vi "Main.vi"(10 "JQMHStartup":refnum<class "ModuleStartup.lvclass">, 11 "SingleLoopTemplate in":refnum<class "Metronome.lvclass">) -> ()   [LabVIEW 2024, in "Metronome.lvclass"]
uses:
  Metronome.lvclass
  C:/Git/JA/JQMH/RQMHCore/ModuleCore/Module.lvclass
  RQMHCore/Startup/ModuleStartup.lvclass
  RQMHCore/ModuleCore/Module.lvclass/Module.ctl
  RQMHCore/ActionStack/Stack/Stack.lvclass/Stack.ctl
  RQMHCore/ActionStack/Stack/Stack.lvclass
  Metronome.lvclass/Metronome.ctl
  C:/Git/JA/JQMH/ModuleTemplates/Metronome/Metronome.lvclass
  RQMHCore/ModuleCore/Module.lvclass
  RQMHCore/ModuleCore/Reply.ctl
  <vilib>/Utility/miscctls.llb/LVPointTypeDef.ctl
  RQMHCore/ModuleCore/InitialiseReplyArgs.ctl
  RQMHCore/ActionStack/Stack/StackFromSingleWithPayload.vi
  RQMHCore/ActionStack/Stack/InitFromString.vi
  RQMHCore/ActionStack/Stack/AppendStacks.vi
  Do Something Args.ctl
panel:
  out "period (ms)":u32
  out "error out":errorcluster
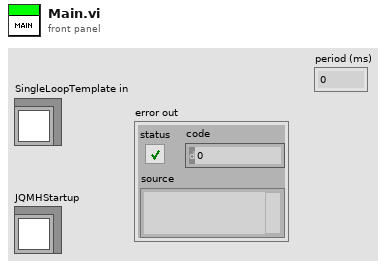
[diagram p1: front panel]
types:
  T1 = typedef "Metronome.lvclass/Request Events--cluster.ctl" = cluster{"Do Something":refnum<user-event>}
  T2 = cluster{"StandardRequests":refnum<event-registration>, "Event Registration Refnum":refnum<event-registration>}
  T3 = cluster{"Module":refnum<class "Metronome.lvclass">, "Args":string}
  T4 = typedef "Module.lvclass/Reply.ctl" = cluster{"Expects Reply":bool, "Reply":refnum<notifier>}
  T5 = enum32{"Invalid", "Standard", "Closed", "Hidden", "Minimized", "Maximized"}
  T6 = typedef "Module.lvclass/InitialiseReplyArgs.ctl" = cluster{"Did Init?":bool}
  T7 = typedef "LVPointTypeDef.ctl" = cluster{"Horizontal":i16, "Vertical":i16}
  T8 = typedef "Metronome.lvclass/Do Something Args.ctl" = cluster{"period (ms)":u32}
  T9 = typedef "JQMHModule.lvclass/Show Front Panel--Args.ctl" = variant
  T10 = typedef "JQMHModule.lvclass/Show Block Diagram.ctl" = bool
  T11 = typedef "JQMHModule.lvclass/Reply.ctl" = cluster{"Expects Reply":bool, "Reply":refnum<notifier>}
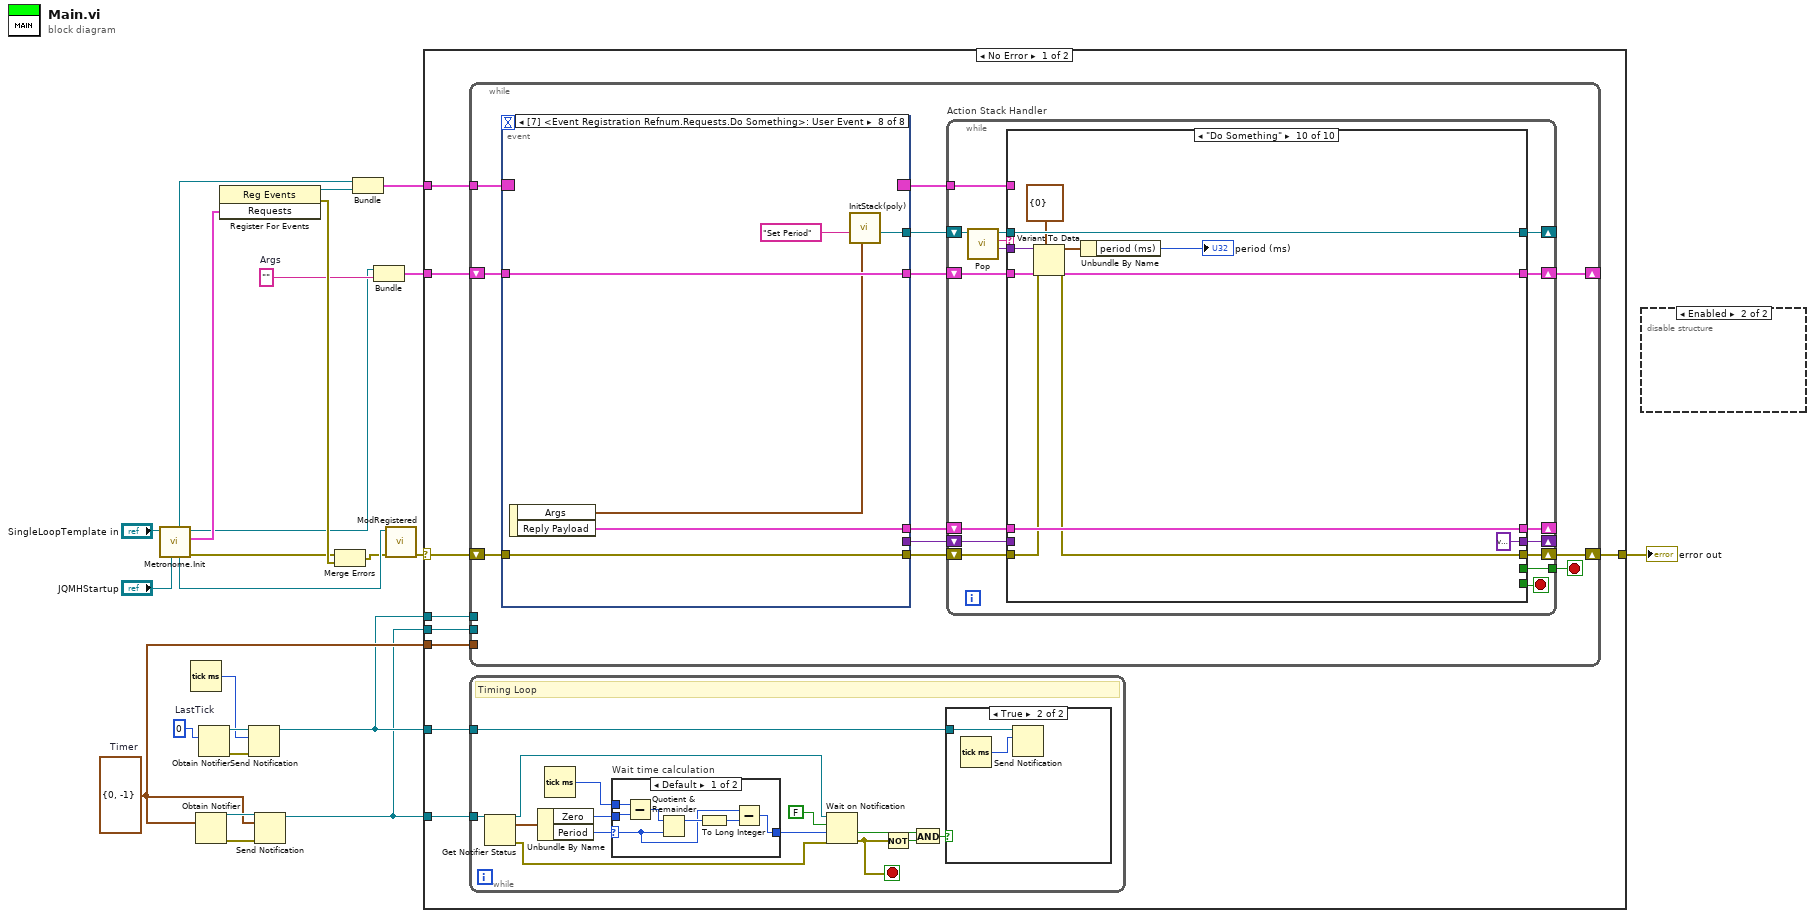
[diagram p0: block diagram]
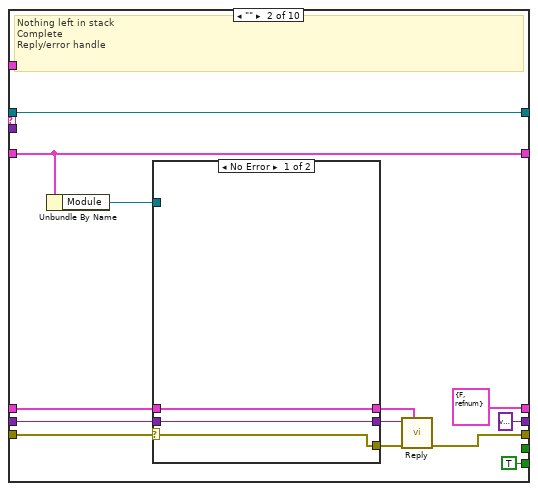
[diagram p3: hidden frame]
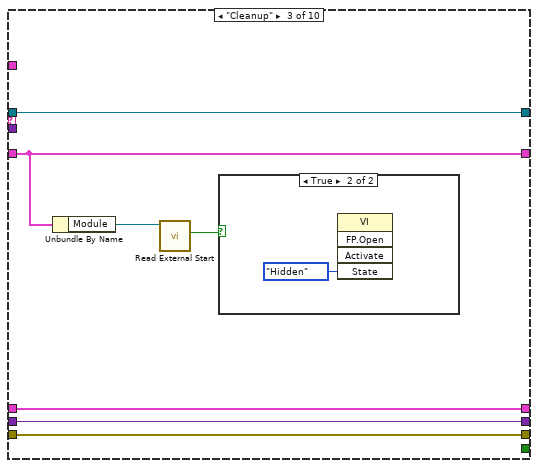
[diagram p5: hidden frame]
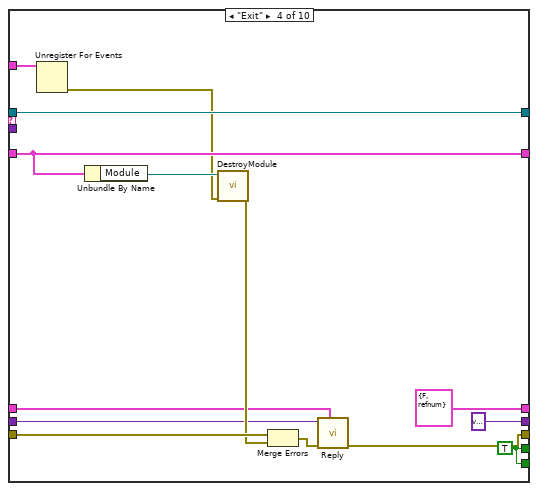
[diagram p7: hidden frame]
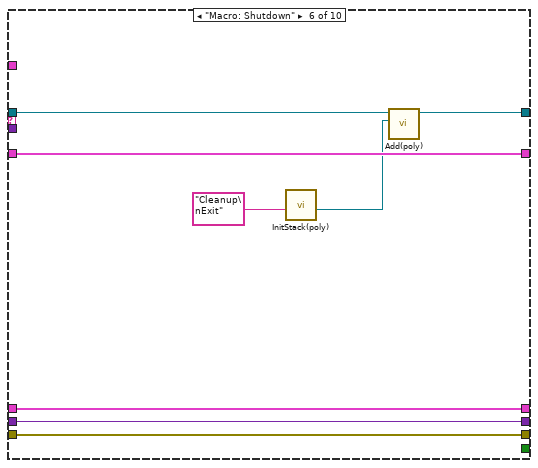
[diagram p9: hidden frame]
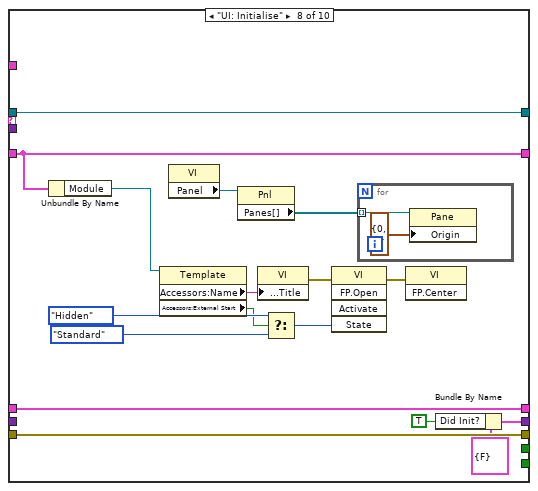
[diagram p11: hidden frame]
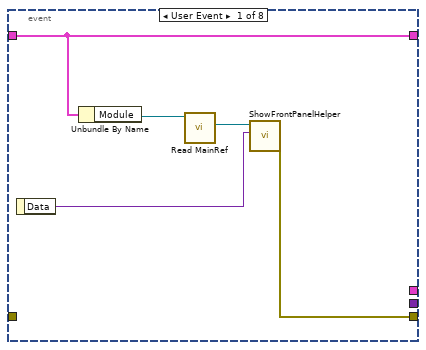
[diagram p13: hidden frame]
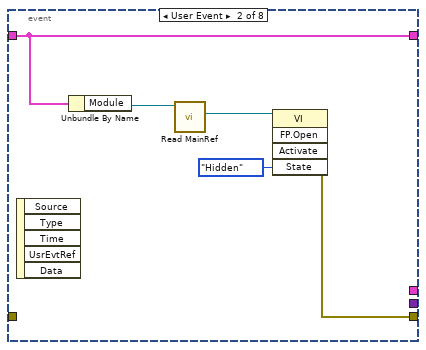
[diagram p14: hidden frame]
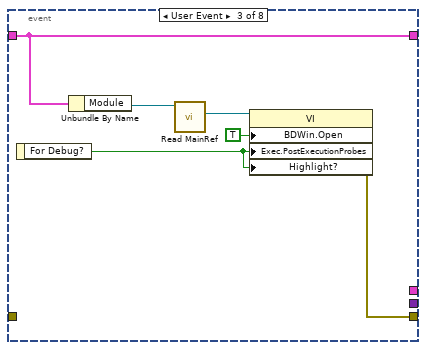
[diagram p15: hidden frame]
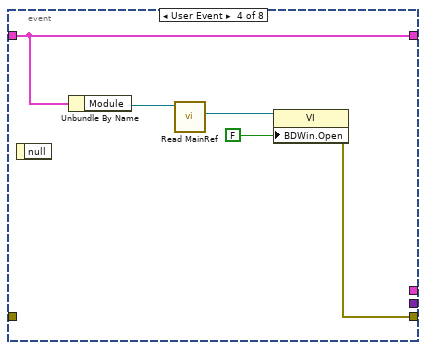
[diagram p16: hidden frame]
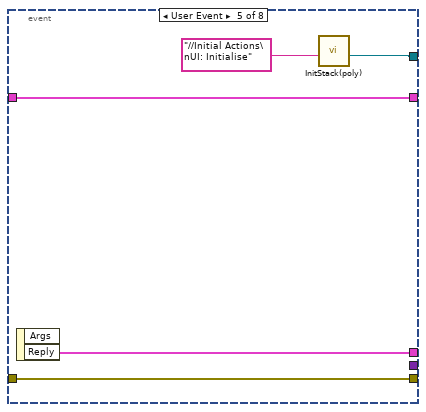
[diagram p17: hidden frame]
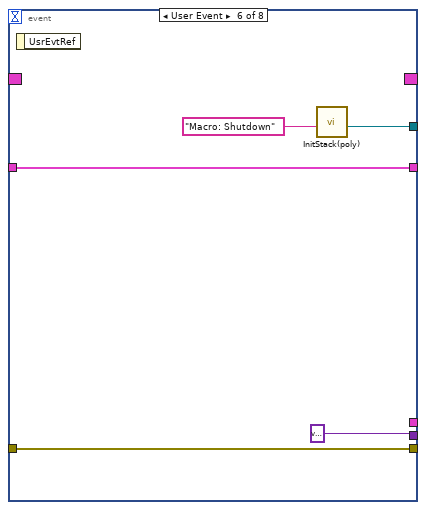
[diagram p18: hidden frame]
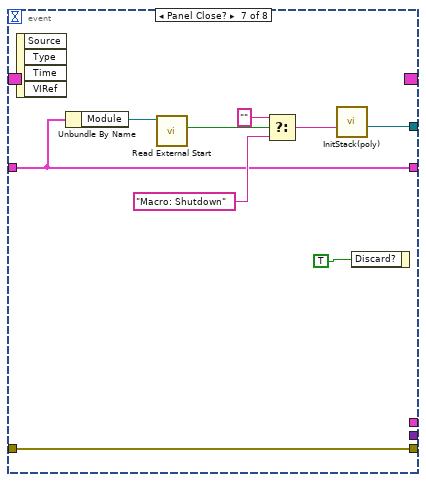
[diagram p19: hidden frame]
diagram:
  w7 = u32 0  # LastTick
  w3 = cluster{"Zero":u32, "Period":i32} {"Zero"=0, "Period"=-1}  # Timer
  w12 = ""  # Args
  n1 = call "Metronome.Init.vi"("JQMHStartup in"="JQMHStartup", "SingleLoopTemplate in"="SingleLoopTemplate in") -> ("error out"=w20:errorcluster, "Requests"=w15:T1, "Module"=w10:refnum<class "Metronome.lvclass">, "JQMHStartup out"=w19:refnum<class "ModuleStartup.lvclass">, "StandardRequests"=w11:refnum<event-registration>)  [unwired: 3 in, 2 out]
  n2 = Tick Count (ms)() -> (millisecond timer value=w6:u32)
  n3 = Obtain Notifier(notification data type=w3) -> (notifier out=w9:refnum<notifier>, error out=w4:errorcluster)  [unwired: 2 in, 2 out]
  n4 = Obtain Notifier(notification data type=w7) -> (notifier out=w8:refnum<notifier>, error out=w5:errorcluster)  [unwired: 2 in, 2 out]
  n5 = register-events(w15) -> (reference out=w16:refnum<event-registration>, error out=w24:errorcluster)  [unwired: 2 in]
  n6 = Send Notification(notification=w6, notifier=w8, error in (no error)=w5) -> (notifier out=w2:refnum<notifier>)  [unwired: 1 out]
  n7 = Send Notification(notification=w3, notifier=w9, error in (no error)=w4) -> (notifier out=w1:refnum<notifier>)  [unwired: 1 out]
  n8 = Merge Errors(w20, w24) -> (w17:errorcluster)
  n9 = Bundle("StandardRequests"=w11, "Event Registration Refnum"=w16) -> (w13:T2)  [unwired: 1 in]
  n10 = Bundle("Module"=w10, "Args"=w12) -> (w14:T3)  [unwired: 1 in]
  n11 = call "ModRegistered.vi"("error in (no error)"=w17, "JQMHStartup in"=w19) -> ("error out"=w18:errorcluster)  [unwired: 9 in]
  n12 = case "RQMH_MAIN" shown="No Error" w18 {
    selector: w18 -> [w32 w233]
    tunnel: w13 -> [w30 w232]
    tunnel: [w33 w233] -> w22
    tunnel: w14 -> [w31 w231]
    tunnel: w1 -> [w29 _]
    tunnel: w2 -> [w28 _]
    tunnel: w3 -> [w27 _]
    tunnel: w2 -> [w26 _]
    tunnel: w1 -> [w25 _]
    frame No Error {
      n13 = while {
        shift-right: [w38] -> w33
        shift-left: w32 -> [w45]
        shift-right: [w40] -> _
        shift-left: w31 -> [w41]
        tunnel: w30 -> [w34]
        tunnel: w27 -> [_]
        tunnel: w26 -> [_]
        tunnel: w25 -> [_]
        stop <- w37 stop-if-true
        n14 = event "RQMH_EVENT_MAIN" shown="[7] <Event Registration Refnum.Requests.Do Something>: User Event" {
          selector: w34 -> [_ _ _ _ _ _ _ _]
          dyn-events: [_ _ _ _ _ _ _ _] -> w44
          timeout: _ -> [_ _ _ _ _ _ _ _]
          tunnel: w45 -> [_ _ _ _ w185 w190 w199 w205]
          tunnel: [w161 w165 w170 w176 w185 w190 w199 w205] -> w39
          tunnel: [_ _ _ _ w181 w186 w192 w200] -> w43
          tunnel: w41 -> [w164 w167 w174 w179 w184 w188 w191 w203]
          tunnel: [w164 w167 w174 w179 w184 w188 w191 w203] -> w42
          tunnel: [_ _ _ _ w183 _ _ w201] -> w36
          tunnel: [_ _ _ _ _ variant _ _] -> w35
          event User Event {
            n15 = event-data() -> ("Data"=w160:T9)  [unwired: 1 in]
            n16 = Unbundle By Name(w164) -> ("Module"=w163:refnum<class "Metronome.lvclass">)
            n17 = call "Read MainRef.vi"("RQMHModule in"=w163) -> ("MainRef"=w162:refnum<vi>)  [unwired: 8 in, 2 out]
            n18 = call "ShowFrontPanelHelper.vi"("Data"=w160, "VI in"=w162) -> ("error out"=w161:errorcluster)  [unwired: 9 in]
          }
          event User Event {
            n19 = event-data() -> ()  [unwired: 1 in, 5 out]
            n20 = Unbundle By Name(w167) -> ("Module"=w168:refnum<class "Metronome.lvclass">)
            n21 = call "Read MainRef.vi"("RQMHModule in"=w168) -> ("MainRef"=w166:refnum<vi>)  [unwired: 8 in, 2 out]
            n22 = invoke class="VI" method="FP.Open"(reference=w166, "State"=T5."Hidden") -> (error out=w165:errorcluster)  [unwired: 3 in, 4 out]
          }
          event User Event {
            n23 = event-data() -> ("For Debug?"=w171:T10)  [unwired: 1 in]
            n24 = Unbundle By Name(w174) -> ("Module"=w175:refnum<class "Metronome.lvclass">)
            n25 = call "Read MainRef.vi"("RQMHModule in"=w175) -> ("MainRef"=w172:refnum<vi>)  [unwired: 8 in, 2 out]
            n26 = property class="VI"(reference=w172, "BDWin.Open"=TRUE ("Block Diagram Window:Open"), "Exec.PostExecutionProbes"=w171, "Highlight?"=w171) -> (error out=w170:errorcluster)  [unwired: 1 in, 1 out]
          }
          event User Event {
            n27 = event-data() -> ()  [unwired: 1 in, 1 out]
            n28 = Unbundle By Name(w179) -> ("Module"=w180:refnum<class "Metronome.lvclass">)
            n29 = call "Read MainRef.vi"("RQMHModule in"=w180) -> ("MainRef"=w177:refnum<vi>)  [unwired: 8 in, 2 out]
            n30 = property class="VI"(reference=w177, "BDWin.Open"=FALSE ("Block Diagram Window:Open")) -> (error out=w176:errorcluster)  [unwired: 1 in, 1 out]
          }
          event User Event {
            n31 = event-data() -> ("Reply"=w183:T11)  [unwired: 1 in, 1 out]
            n32 = call-poly "InitStack(poly).vi"("ActionStack String"="//Initial Actions\nUI: Initialise") -> ("ActionStack out"=w181:refnum<class "Stack.lvclass">)  [unwired: 10 in]
          }
          event User Event {
            (unwired) errorcluster {"status"=FALSE, "code"=0, "source"=""} ("error out")
            (unwired) TRUE
            n33 = event-data() -> ()  [unwired: 1 in, 1 out]
            n34 = call-poly "InitStack(poly).vi"("Action"="Macro: Shutdown") -> ("Stack out"=w186:refnum<class "Stack.lvclass">)  [unwired: 10 in]
          }
          event Panel Close? {
            n35 = event-data() -> ()  [unwired: 1 in, 4 out]
            n36 = Unbundle By Name(w191) -> ("Module"=w197:refnum<class "Metronome.lvclass">)
            n37 = call "Read External Start.vi"("JQMHModule in"=w197) -> ("External Start?"=w196:bool)  [unwired: 8 in, 2 out]
            n38 = Select(t="", s=w196, f="Macro: Shutdown" ("Action")) -> (s? t:f=w193:string)
            n39 = call-poly "InitStack(poly).vi"("Action"=w193) -> ("Stack out"=w192:refnum<class "Stack.lvclass">)  [unwired: 10 in]
            n40 = event-data("Discard?"=TRUE) -> ()  [unwired: 1 in, 1 out]
          }
          event User Event {
            n41 = event-data() -> ("Args"=w202:T8, "Reply Payload"=w201:T4)  [unwired: 1 in]
            n42 = call-poly "InitStack(poly).vi"("Payload"=w202, "Action"="Set Period" ("Message")) -> ("Stack out"=w200:refnum<class "Stack.lvclass">)  [unwired: 9 in]
          }
        }
        n43 = while "Action Stack Handler" {
          shift-right: [w61] -> _
          shift-left: w43 -> [w53]
          shift-right: [w58] -> w38
          shift-left: w39 -> [w59]
          tunnel: w44 -> [w57]
          shift-right: [w55] -> w40
          shift-left: w42 -> [w56]
          tunnel: [w54] -> w37
          shift-right: [w48] -> _
          shift-left: w36 -> [w49]
          shift-right: [w47] -> _
          shift-left: w35 -> [w46]
          stop <- w60 stop-if-true
          n44 = call "Pop.vi"("Stack in"=w53) -> ("Popped Payload"=w50:variant, "Popped Action"=w51:string, "Stack out"=w52:refnum<class "Stack.lvclass">)  [unwired: 8 in]
          n45 = case shown="\"Do Something\"" w51 {
            tunnel: w52 -> [w66 w79 w92 w107 w112 w114 w125 w142 w149 w159]
            tunnel: [w66 w79 w92 w107 w112 w117 w125 w142 w149 w159] -> w61
            tunnel: w50 -> [_ _ _ _ _ _ _ _ _ w156]
            tunnel: [_ TRUE ("Boolean") _ w105 _ _ _ _ _ _] -> w60
            tunnel: w59 -> [w62 w77 w91 w99 w110 w119 w124 w141 w148 w153]
            tunnel: [w62 w72 w91 w94 w110 w119 w124 w141 w148 w154] -> w58
            tunnel: w57 -> [_ _ _ w106 _ _ _ _ _ _]
            tunnel: w56 -> [w65 w76 w86 w101 w111 w120 w123 w138 w147 w158]
            tunnel: [w65 w76 w86 w101 w111 w120 w123 w138 w147 w158] -> w55
            tunnel: [_ _ _ w105 _ _ _ _ _ _] -> w54
            tunnel: w49 -> [w64 w73 w90 w95 w109 w116 w122 w140 w146 w157]
            tunnel: [w64 T4 {"Expects Reply"=FALSE, "Reply"=refnum} ("Reply Payload") w90 T4 {"Expects Reply"=FALSE, "Reply"=refnum} ("Reply Payload") w109 w116 w122 w140 w146 w157] -> w48
            tunnel: [w63 variant ("Variant") w89 variant ("Variant") w108 w115 w121 w133 w145 variant ("Variant")] -> w47
            tunnel: w46 -> [w63 w68 w89 w96 w108 w115 w121 _ w145 _]
            frame Default {
              # "#TODO Add Error Handling"
            }
            frame "" {
              # "Nothing left in stack\nComplete\nReply/error handle"
              n46 = Unbundle By Name(w76) -> ("Module"=w75:refnum<class "Metronome.lvclass">)
              n47 = case shown="No Error" w77 {
                selector: w77 -> [w80 w84]
                tunnel: [w82 w85] -> w74
                tunnel: w73 -> [w82 w85]
                tunnel: [w81 w83] -> w69
                tunnel: w68 -> [w81 w83]
                tunnel: w75 -> [_ _]
                tunnel: [w80 w84] -> w67
                frame No Error {
                }
                frame Error {
                }
              }
              n48 = call "Reply.vi"("Reply"=w74, "error in (no error)"=w67, "ReplyPayload"=w69) -> ("error out"=w72:errorcluster)  [unwired: 8 in]
            }
            frame "Cleanup" {
              n49 = Unbundle By Name(w86) -> ("Module"=w88:refnum<class "Metronome.lvclass">)
              n50 = call "Read External Start.vi"("JQMHModule in"=w88) -> ("External Start?"=w87:bool)  [unwired: 8 in, 2 out]
              n51 = case shown="True" w87 {
                frame False {
                }
                frame True {
                  n52 = invoke class="VI" method="FP.Open"("State"=T5."Hidden") -> ()  [unwired: 4 in, 5 out]
                }
              }
            }
            frame "Exit" {
              w105 = TRUE
              n53 = Unregister For Events(event registration refnum=w106) -> (error out=w100:errorcluster)  [unwired: 1 in]
              n54 = Unbundle By Name(w101) -> ("Module"=w102:refnum<class "Metronome.lvclass">)
              n55 = call "DestroyModule.vi"("error in (no error)"=w100, "JQMHModule in"=w102) -> ("error out"=w98:errorcluster)  [unwired: 9 in]
              n56 = Merge Errors(w99, w98) -> (w97:errorcluster)
              n57 = call "Reply.vi"("Reply"=w95, "error in (no error)"=w97, "ReplyPayload"=w96) -> ("error out"=w94:errorcluster)  [unwired: 8 in]
            }
            frame "---------- Macros ----------" {
            }
            frame "Macro: Shutdown" {
              n58 = call-poly "InitStack(poly).vi"("ActionStack String"="Cleanup\nExit") -> ("ActionStack out"=w113:refnum<class "Stack.lvclass">)  [unwired: 10 in]
              n59 = call-poly "Add(poly).vi"("Second"=w113, "First"=w114) -> ("First"=w117:refnum<class "Stack.lvclass">)  [unwired: 9 in]
            }
            frame "---------- UI ----------" {
              # "Add module specific commands"
            }
            frame "UI: Initialise" {
              n60 = Unbundle By Name(w138) -> ("Module"=w137:refnum<class "Metronome.lvclass">)
              n61 = property class="Template"(reference=w137) -> ("Accessors:Name"=w128:string, "Accessors:External Start"=w127:bool)  [unwired: 1 in, 2 out]
              n62 = property on="Property Node" class="VI"() -> ("Panel"=w130:refnum<vi>)  [unwired: 2 in, 2 out]
              n63 = property on="Property Node" class="Pnl"(reference=w130) -> ("Panes[]"=w129:refnum<vi>[])  [unwired: 1 in, 2 out]
              n64 = property on="Property Node" class="VI"("Front Panel.Title"=w128) -> (error out=w132:errorcluster)  [unwired: 2 in, 1 out]
              n65 = Select(t=T5."Hidden" ("State"), s=w127, f=T5."Standard" ("State")) -> (s? t:f=w126:T5)
              n66 = invoke on="Invoke Node" class="VI" method="FP.Open"(error in=w132, "State"=w126) -> (error out=w131:errorcluster)  [unwired: 3 in, 4 out]
              n67 = for {
                tunnel: w129 -> [w143] mode=indexing
                n68 = property on="Property Node" class="Pane"(reference=w143, "Origin"=T7 {"Horizontal"=0, "Vertical"=0}) -> ()  [unwired: 1 in, 2 out]
              }
              n69 = invoke on="Invoke Node" class="VI" method="FP.Center"(error in=w131) -> ()  [unwired: 2 in, 3 out]
              n70 = Bundle By Name(cluster=T6 {"Did Init?"=FALSE} ("Args"), "Did Init?"=TRUE) -> (w133:T6)
            }
            frame "---------- Actions ----------" {
              # "Add module specific commands"
            }
            frame "Do Something" {
              n71 = Variant To Data(error in=w153, type=T8 {"period (ms)"=0} ("Args"), Variant=w156) -> (data=w152:T8, error out=w154:errorcluster)
              n72 = Unbundle By Name(w152) -> ("period (ms)"=→"period (ms)":u32)
            }
          }
        }
      }
      n73 = while "\"Ticker\" Loop" {
        tunnel: w29 -> [w214]
        tunnel: w28 -> [w206]
        stop <- w208 stop-if-true
        # "Timing Loop"
        n74 = Get Notifier Status(notifier=w214) -> (notifier out=w213:refnum<notifier>, current notification=w212:cluster{"Zero":u32, "Period":i32}, error out=w210:errorcluster)  [unwired: 1 in, 2 out]
        n75 = Unbundle By Name(w212) -> ("Zero"=w219:u32, "Period"=w217:i32)
        n76 = Tick Count (ms)() -> (millisecond timer value=w218:u32)
        n77 = case "Wait time calculation" shown="Default" w217 {
          selector: w217 -> [w220 w227]
          tunnel: [w222 w227] -> w211
          tunnel: w219 -> [w226 _]
          tunnel: w218 -> [w225 _]
          frame Default {
            n78 = Subtract(x=w225, y=w226) -> (x-y=w224:u32)
            n79 = Quotient & Remainder(x=w224, y=w220) -> (x-y*floor(x/y)=w223:u32)  [unwired: 1 out]
            n80 = To Long Integer(number=w223) -> (32bit integer=w221:i32)
            n81 = Subtract(x=w220, y=w221) -> (x-y=w222:i32)
          }
          frame -1 {
          }
        }
        n82 = Wait on Notification(notifier=w213, ignore previous (F)=FALSE, timeout in ms (-1)=w211, error in (no error)=w210) -> (timed out?=w215:bool, error out=w208:errorcluster)  [unwired: 2 out]
        n83 = Not(x=w208) -> (.not. x?=w207:bool)
        n84 = And(x=w215, y=w207) -> (x .and. y?=w209:bool)
        n85 = case "Tick" shown="True" w209 {
          tunnel: w206 -> [_ w229]
          frame False {
          }
          frame True {
            n86 = Tick Count (ms)() -> (millisecond timer value=w228:u32)
            n87 = Send Notification(notification=w228, notifier=w229) -> ()  [unwired: 1 in, 2 out]
          }
        }
      }
    }
    frame Error {
      n88 = Unregister For Events(event registration refnum=w232) -> ()  [unwired: 1 in, 1 out]
      n89 = Unbundle(w231) -> ("Module"=w230:refnum<class "Metronome.lvclass">)  [unwired: 1 out]
      n90 = call "DestroyModule.vi"("JQMHModule in"=w230) -> ()  [unwired: 10 in, 1 out]
    }
  }
  "error out" <- w22
  n91 = disable-structure shown="Enabled" {
    frame Disabled {
    }
    frame Enabled {
    }
  }
